vi "Test MQTT-3.6.1-1.vi"(8 "error in (no error)":errorcluster) -> (0 "error out":errorcluster)   [LabVIEW 2013]
uses:
  <vilib>/LabVIEW Open Source Project/MQTT Control Packets/Control Packets/ControlPacket/ControlPacket.lvclass/ControlPacket.ctl
  <vilib>/addons/_JKI Toolkits/Caraya/classes/Test/Test.lvclass
  <vilib>/LabVIEW Open Source Project/MQTT Control Packets/Control Packets/PUBREL/PUBREL.lvclass
  <vilib>/LabVIEW Open Source Project/MQTT Control Packets/Control Packets/ControlPacket/ControlPacket.lvclass
  <vilib>/addons/_JKI Toolkits/Caraya/classes/Assert/Assert.lvclass
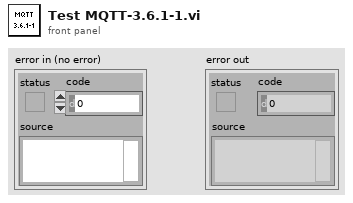
[diagram p1: front panel]
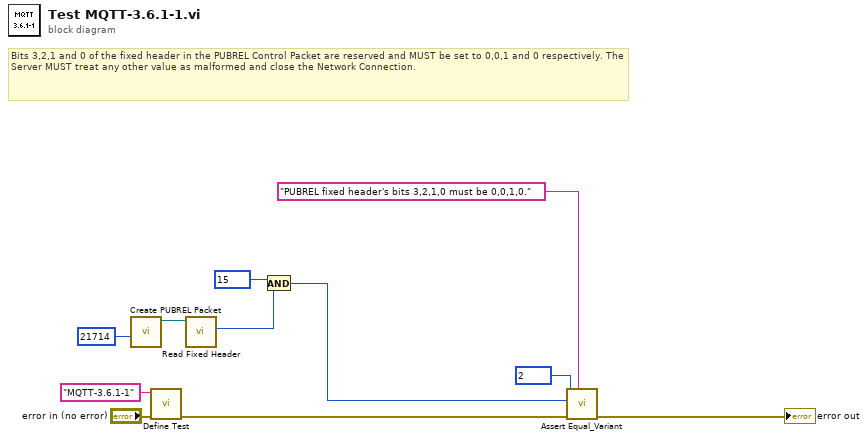
[diagram p0: block diagram]
diagram:
  # "Bits 3,2,1 and 0 of the fixed header in the PUBREL Control Packet are reserved and MUST be set to 0,0,1 and 0 respectively. The Server MUST treat any other value as malformed and close the Network Connection."
  n1 = call <vilib>:"Create PUBREL Packet.vi"("Packet ID"=u16 21714) -> ("PUBREL out"=w5:refnum<class "PUBREL.lvclass">)  [unwired: 8 in, 2 out]
  n2 = call <vilib>:"Define Test.vi"("error in (no error)"="error in (no error)", "Label (VI Title)"="MQTT-3.6.1-1") -> ("error out"=w8:errorcluster)  [unwired: 9 in]
  n3 = call <vilib>:"Read Fixed Header.vi"("ControlPacket in"=w5) -> ("Fixed Header"=w4:u8)  [unwired: 9 in, 1 out]
  n4 = And(x=u8 15, y=w4) -> (x .and. y?=w1:u8)
  n5 = call <vilib>:"Assert Equal_Variant.vi"("Label"="PUBREL fixed header's bits 3,2,1,0 must be 0,0,1,0.", "error in (no error)"=w8, "Y"=w1, "X"=u8 2 ("x")) -> ("error out"=→"error out":errorcluster)  [unwired: 7 in]
